vi "OutcomeStringToBool.vi"(11 "outcome string":string) -> (3 "outcome bool":bool)   [LabVIEW 2019, in "ByteQXWebAPI.lvlib" / "ByteQXAPIBase.lvclass"]
doc: "Convers a String to True or False based on \"P\" or \"F\""
uses:
  ByteQXAPIBase.lvclass
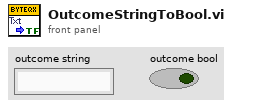
[diagram p1: front panel]
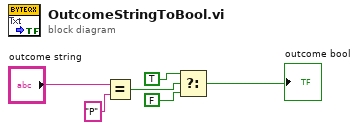
[diagram p0: block diagram]
diagram:
  n1 = Equal?(x="outcome string", y="P") -> (x = y?=w4:bool)
  n2 = Select(t=TRUE, s=w4, f=FALSE) -> (s? t:f=→"outcome bool":bool)
